vi "ExeVersionInformation_LV2010SP1.vi"() -> ()   [LabVIEW 2012]
panel:
  out "FileVersion":string
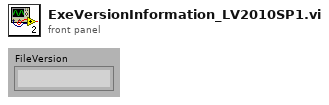
[diagram p1: front panel]
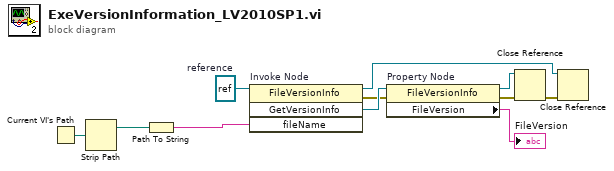
[diagram p0: block diagram]
diagram:
  w11 = refnum<k24> refnum  # reference
  n1 = Current VI's Path() -> (path=w10:path)
  n2 = Strip Path(path=w10) -> (stripped path=w9:path)  [unwired: 1 out]
  n3 = Path To String(path=w9) -> (string=w8:string)
  n4 = invoke on="Invoke Node" class="FileVersionInfo" method="GetVersionInfo"(reference=w11, "fileName"=w8) -> (reference out=w1:refnum<k24>, error out=w6:errorcluster, "GetVersionInfo"=w7:refnum<k24>)  [unwired: 2 in, 1 out]
  n5 = property on="Property Node" class="FileVersionInfo"(reference=w7, error in=w6) -> (reference out=w4:refnum<k24>, error out=w3:errorcluster, "FileVersion"=→"FileVersion":string)
  n6 = Close Reference(reference=w4, error in (no error)=w3) -> (error out=w2:errorcluster)
  n7 = Close Reference(reference=w1, error in (no error)=w2) -> ()  [unwired: 1 out]
